vi "Configure Filter.vi"(0 "VISA resource name":refnum<visa-resource-name>, 1 "Function (0: Volts)":u16(ring) items=["Volts", "Current", "Resistance"], 2 "Enable Filter  (T: Enable)":bool=TRUE, 3 "Filter Type  (0: Repeating)":u16(ring) items=["Repeating", "Moving"], 4 "Number of Filter Readings (3)":u32=10 min=1 max=100 step=1, 5 "error in (no error)":errorcluster) -> (14 "VISA resource name out":refnum<visa-resource-name>, 19 "error out":errorcluster)   [LabVIEW 2022 SP3, in "Keithley 2450.lvlib"]
doc: "Configures the measurement filter, including the number of readings averaged the type of filter applied."
uses:
  Keithley 2450.lvlib
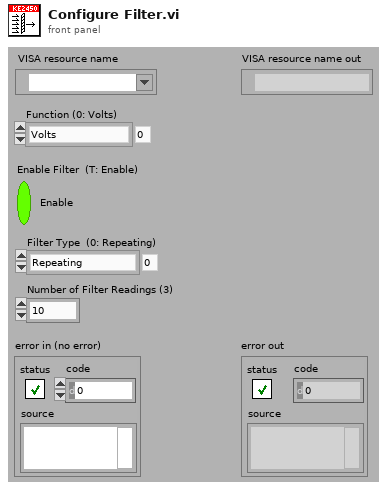
[diagram p1: front panel]
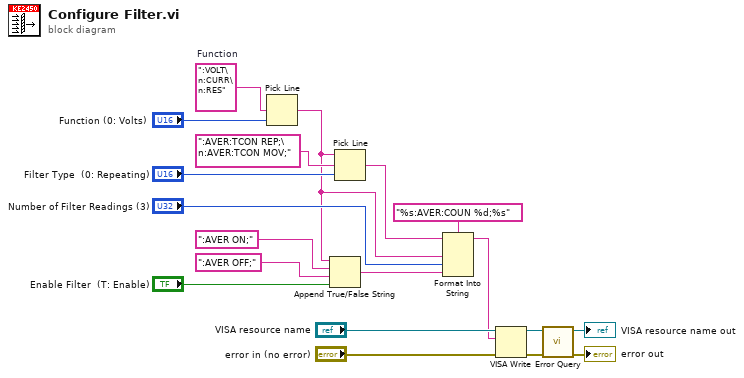
[diagram p0: block diagram]
diagram:
  w9 = ":VOLT\n:CURR\n:RES"  # Function
  n1 = Pick Line(multi-line string=w9, line index="Function (0: Volts)") -> (output string=w2:string)  [unwired: 1 out]
  n2 = Append True/False String(1:"Enable Filter  (T: Enable)", 2:":AVER OFF;", 3:":AVER ON;", 4:w2) -> (0:w4:string)
  n3 = Pick Line(string ("")=w2, multi-line string=":AVER:TCON REP;\n:AVER:TCON MOV;", line index="Filter Type  (0: Repeating)") -> (output string=w1:string)
  n4 = Format Into String(format string="%s:AVER:COUN %d;%s", initial string=w1, w2, "Number of Filter Readings (3)", w4) -> (resulting string=w10:string)  [unwired: 1 in, 1 out]
  n5 = VISA Write(VISA resource name="VISA resource name", write buffer=w10, error in (no error)="error in (no error)") -> (VISA resource name out=w15:refnum<visa-resource-name>, error out=w14:errorcluster)  [unwired: 1 out]
  n6 = call "Error Query.vi"("error in (no error)"=w14, "VISA resource name"=w15) -> ("error out"=→"error out":errorcluster, "VISA resource name out"=→"VISA resource name out":refnum<visa-resource-name>)  [unwired: 8 out]
